vi "BRig_Host__Loop_Consumer_RunState__typeTrial__getSubType.vi"(11 "input_strCmd":string) -> (2 "output_Trial_subtype":u8)   [LabVIEW 2014]
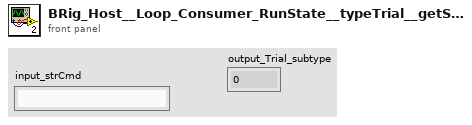
[diagram p1: front panel]
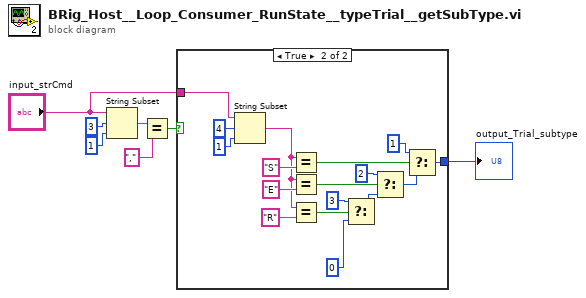
[diagram p0: block diagram]
diagram:
  n1 = String Subset(string="input_strCmd", offset (0)=3, length (rest)=1 ("offset (0)")) -> (substring=w3:string)
  n2 = Equal?(x=w3, y=",") -> (x = y?=w2:bool)
  n3 = case shown="True" w2 {
    tunnel: "input_strCmd" -> [_ w23]
    tunnel: [_ w14] -> w6
    frame False {
    }
    frame True {
      n4 = String Subset(string=w23, offset (0)=4, length (rest)=1 ("offset (0)")) -> (substring=w12:string)
      n5 = Equal?(x=w12, y="S") -> (x = y?=w16:bool)
      n6 = Equal?(x=w12, y="E") -> (x = y?=w19:bool)
      n7 = Equal?(x=w12, y="R") -> (x = y?=w10:bool)
      n8 = Select(t=u8 3, s=w10, f=u8 0 ("offset (0)")) -> (s? t:f=w9:u8)
      n9 = Select(t=u8 2, s=w19, f=w9) -> (s? t:f=w15:u8)
      n10 = Select(t=u8 1, s=w16, f=w15) -> (s? t:f=w14:u8)
    }
  }
  "output_Trial_subtype" <- w6
